vi "TCS_Ctrl_=.vi"(0 "VRN IN":refnum<visa-resource-name>="-1", 2 "Commande #":i32=-1, 7 "Args":dbl[](array[numeric]) format="%.2f", 11 "Error IN":errorcluster) -> (4 "VRN OUT":refnum<visa-resource-name>="-1", 8 "OK Done":bool, 15 "Error OUT":errorcluster)   [LabVIEW 2011]
panel:
  out "Cmd String":string
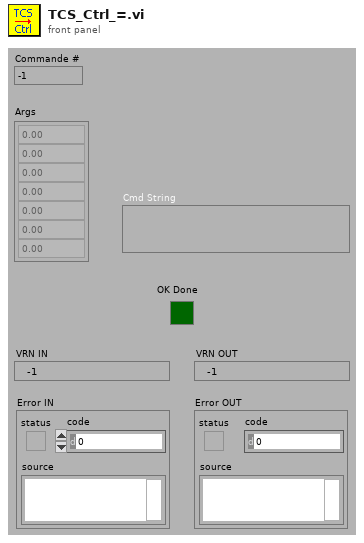
[diagram p1: front panel]
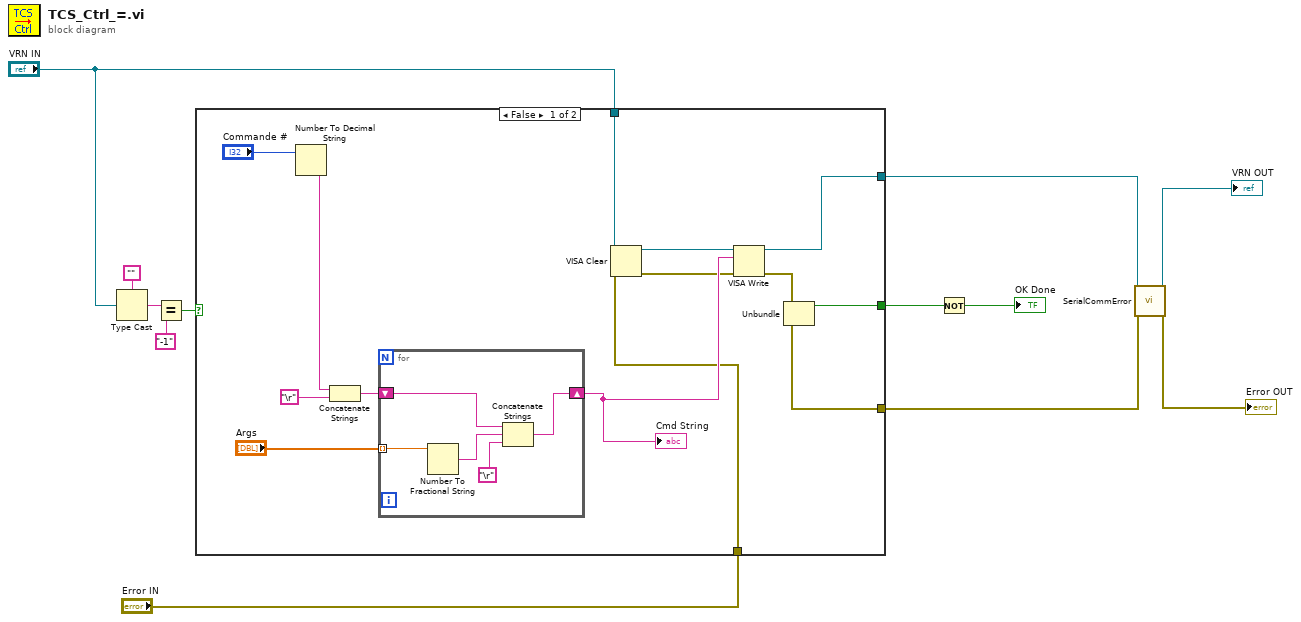
[diagram p0: block diagram]
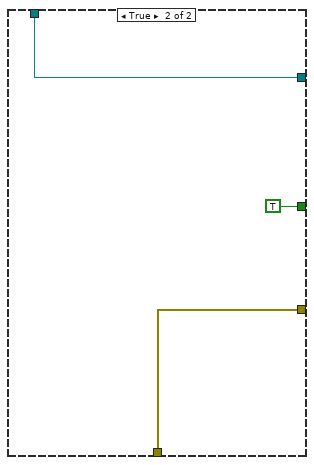
[diagram p2: hidden frame]
diagram:
  n1 = Type Cast(type="", x="VRN IN") -> (*(type *) &x=w9:string)
  n2 = Equal?(x=w9, y="-1") -> (x = y?=w7:bool)
  n3 = case shown="False" w7 {
    tunnel: [w24 TRUE ("status")] -> w11
    tunnel: "VRN IN" -> [w15 w31]
    tunnel: [w22 w32] -> w3
    tunnel: "Error IN" -> [w16 w32]
    tunnel: [w17 w31] -> w4
    frame False {
      n4 = Number To Decimal String(number="Commande #") -> (decimal integer string=w19:string)  [unwired: 1 in]
      n5 = Concatenate Strings(w19, "\r") -> (w20:string)
      n6 = for {
        shift-right: [w28] -> w23
        shift-left: w20 -> [w30]
        tunnel: "Args" -> [w27] mode=indexing
        n7 = Number To Fractional String(number=w27) -> (F-format string=w26:string)  [unwired: 3 in]
        n8 = Concatenate Strings(w30, w26, "\r") -> (w28:string)
      }
      "Cmd String" <- w23
      n9 = VISA Clear(VISA resource name=w15, error in (no error)=w16) -> (VISA resource name out=w14:refnum<visa-resource-name>, error out=w13:errorcluster)
      n10 = VISA Write(VISA resource name=w14, write buffer=w23, error in (no error)=w13) -> (VISA resource name out=w17:refnum<visa-resource-name>, error out=w22:errorcluster)  [unwired: 1 out]
      n11 = Unbundle(w22) -> ("status"=w24:bool)  [unwired: 2 out]
    }
    frame True {
    }
  }
  n12 = Not(x=w11) -> (.not. x?=→"OK Done":bool)
  n13 = call "SerialCommError.vi"("VISA IN"=w4, "error IN"=w3) -> ("VISA OUT"=→"VRN OUT":refnum<visa-resource-name>, "error OUT"=→"Error OUT":errorcluster)  [unwired: 11 in, 1 out]
